vi "Frame Set c.vi"(8 "error in (no error)":errorcluster, 10 "<c> Data":T1, 11 "IDE simple in":refnum<class "Main Panel.lvclass">) -> (0 "error out":errorcluster, 3 "IDE simple out":refnum<class "Main Panel.lvclass">)   [LabVIEW 2018, in "Main Panel.lvlib" / "Main Panel.lvclass"]
uses:
  Main Panel.lvclass
  Frame Analizer/frame c data.ctl
  Main Panel.lvclass/Main Panel.ctl
  Frame Analizer/Data Parser.lvclass
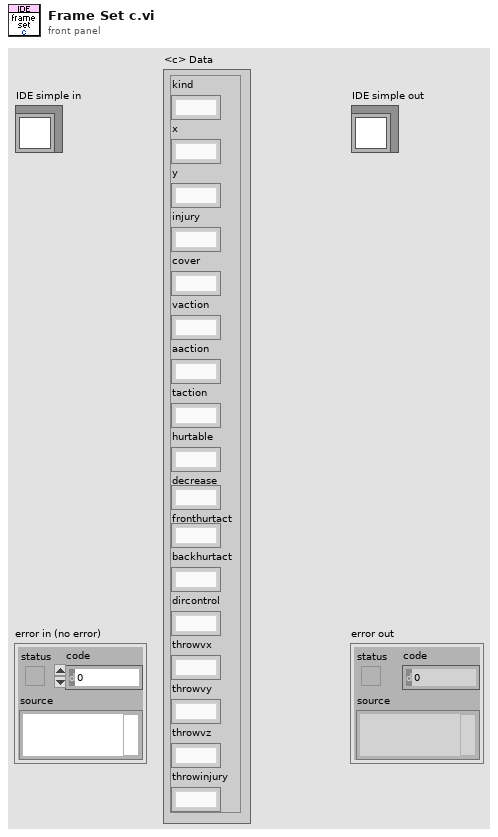
[diagram p1: front panel]
types:
  T1 = typedef "Data Parser.lvclass/frame c data.ctl" = cluster{"kind":string, "x":string, "y":string, "injury":string, "cover":string, "vaction":string, "aaction":string, "taction":string, "hurtable":string, "decrease":string, "fronthurtact":string, "backhurtact":string, "dircontrol":string, "throwvx":string, "throwvy":string, "throwvz":string, "throwinjury":string}
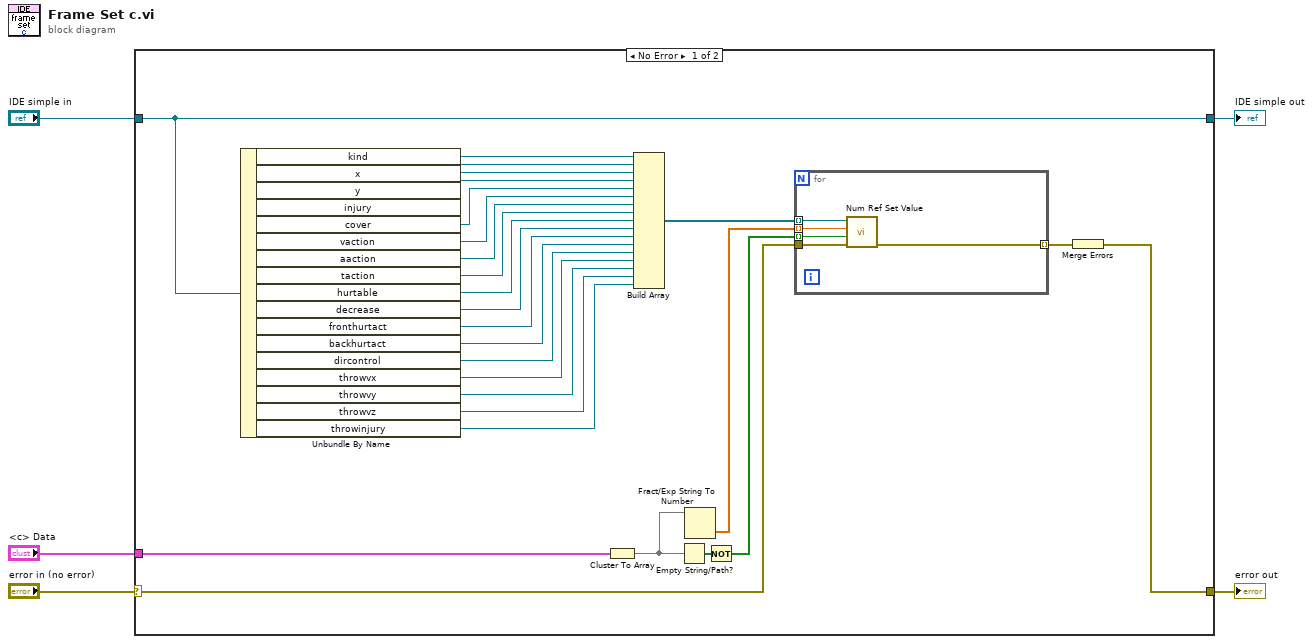
[diagram p0: block diagram]
diagram:
  n1 = case shown="No Error" "error in (no error)" {
    selector: "error in (no error)" -> [w31 w39]
    tunnel: [w26 w39] -> w4
    tunnel: [w28 w38] -> w2
    tunnel: "IDE simple in" -> [w28 w38]
    tunnel: "<c> Data" -> [w25 _]
    frame No Error {
      n2 = Unbundle By Name(w28) -> ("kind"=w22:refnum<vi>, "x"=w21:refnum<vi>, "y"=w20:refnum<vi>, "injury"=w7:refnum<vi>, "cover"=w6:refnum<vi>, "vaction"=w19:refnum<vi>, "aaction"=w18:refnum<vi>, "taction"=w17:refnum<vi>, "hurtable"=w16:refnum<vi>, "decrease"=w15:refnum<vi>, "fronthurtact"=w14:refnum<vi>, "backhurtact"=w13:refnum<vi>, "dircontrol"=w12:refnum<vi>, "throwvx"=w11:refnum<vi>, "throwvy"=w10:refnum<vi>, "throwvz"=w9:refnum<vi>, "throwinjury"=w8:refnum<vi>)
      n3 = Cluster To Array(cluster=w25) -> (array=w24:string[])
      n4 = Build Array(w22, w21, w20, w7, w6, w19, w18, w17, w16, w15, w14, w13, w12, w11, w10, w9, w8) -> (w23:refnum<vi>[])
      n5 = Empty String/Path?(string/path=w24) -> (empty?=w32:bool[])
      n6 = Fract/Exp String To Number(string=w24) -> (number=w29:dbl[])  [unwired: 3 in, 1 out]
      n7 = Not(x=w32) -> (.not. x?=w30:bool[])
      n8 = for {
        tunnel: w31 -> [w37]
        tunnel: w23 -> [w33] mode=indexing
        tunnel: w30 -> [w34] mode=indexing
        tunnel: w29 -> [w36] mode=indexing
        tunnel: [w35] -> w27 mode=indexing
        n9 = call "Num Ref Set Value.vi"("error in"=w37, "Valid"=w34, "Value"=w36, "Num Ref"=w33) -> ("error out"=w35:errorcluster)  [unwired: 7 in]
      }
      n10 = Merge Errors(w27) -> (w26:errorcluster)
    }
    frame Error {
    }
  }
  "error out" <- w4
  "IDE simple out" <- w2
